vi "Host - Firmware Download.vi"(7 "Need Reset":bool, 8 "error in (no error)":errorcluster, 9 "File Byte Array":u8[](array[numeric]), 10 "Firmware filename":path, 11 "Slave Ref in":refnum<k21>) -> (0 "error out":errorcluster)   [LabVIEW 2016, in "Scan Engine Custom Device.lvlib"]
uses:
  Scan Engine Custom Device.lvlib
  <resource>/objmgr/IndComECAT.rc
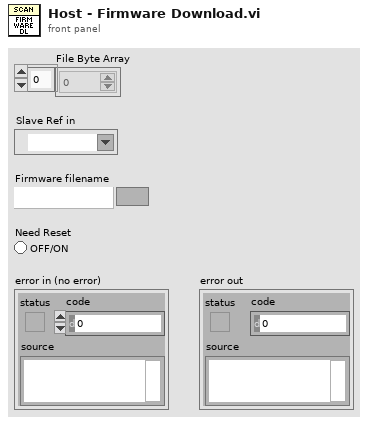
[diagram p1: front panel]
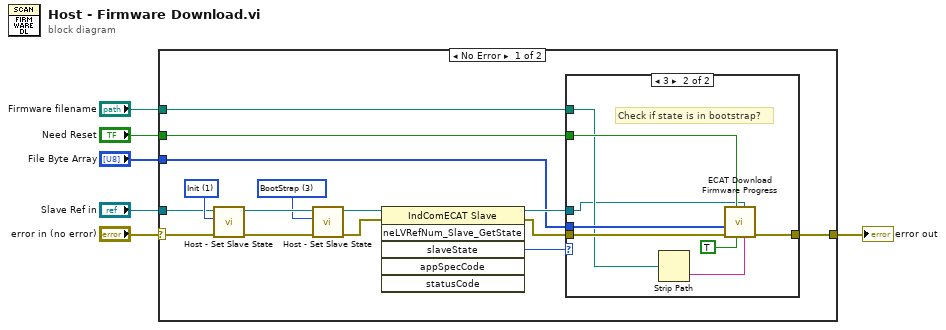
[diagram p0: block diagram]
diagram:
  n1 = case shown="No Error" "error in (no error)" {
    selector: "error in (no error)" -> [w14 w31]
    tunnel: "Slave Ref in" -> [w12 _]
    tunnel: "Need Reset" -> [w20 _]
    tunnel: "File Byte Array" -> [w18 _]
    tunnel: [w16 w31] -> w1
    tunnel: "Firmware filename" -> [w15 _]
    frame No Error {
      w9 = u32 3 items=["Init"=1, "PreOP"=2, "BootStrap"=3, "SafeOP"=4, "OP"=8] ("slaveState")
      w13 = u32 1 items=["Init"=1, "PreOP"=2, "BootStrap"=3, "SafeOP"=4, "OP"=8] ("slaveState")
      n2 = call "Host - Set Slave State.vi"("error in (no error)"=w14, "slaveState"=w13, "Slave Ref in"=w12) -> ("error out"=w11:errorcluster, "Slave Ref out"=w10:refnum<k21>)  [unwired: 5 in, 2 out]
      n3 = call "Host - Set Slave State.vi"("error in (no error)"=w11, "slaveState"=w9, "Slave Ref in"=w10) -> ("error out"=w7:errorcluster, "Slave Ref out"=w8:refnum<k21>)  [unwired: 5 in, 2 out]
      n4 = invoke class="IndComECAT Slave" method="neLVRefNum_Slave_GetState"(reference=w8, error in=w7) -> (reference out=w21:refnum<k21>, error out=w17:errorcluster, "slaveState"=w19:u32)  [unwired: 4 in, 3 out]
      n5 = case shown="3" w19 {
        tunnel: [w22 w28] -> w16
        tunnel: w21 -> [_ w23]
        tunnel: w17 -> [w22 w30]
        tunnel: w18 -> [_ w29]
        tunnel: w20 -> [_ w27]
        tunnel: w15 -> [_ w25]
        frame 0, Default {
        }
        frame 3 {
          # "Check if state is in bootstrap?"
          n6 = Strip Path(path=w25) -> (name=w24:string)  [unwired: 1 out]
          n7 = call "ECAT Download Firmware Progress.vi"("Device Filename"=w24, "Slave Ref"=w23, "ShowFront?"=TRUE, "NeedReset"=w27, "error in"=w30, "File Byte Array"=w29) -> ("Error Out"=w28:errorcluster)  [unwired: 2 in, 3 out]
        }
      }
    }
    frame Error {
    }
  }
  "error out" <- w1
